vi "Get Test Skipped Message.vi"(8 "error in":errorcluster, 11 "Test In":refnum<class>) -> (0 "error out":errorcluster, 1 "IsTestCase":bool, 2 "skipMessage":string, 3 "Test Out":refnum<class>)   [LabVIEW 2013, in "TestResult.lvclass"]
uses:
  TestResult.lvclass
  TestCase/TestCase.lvclass
  TestSuite/TestSuite.lvclass
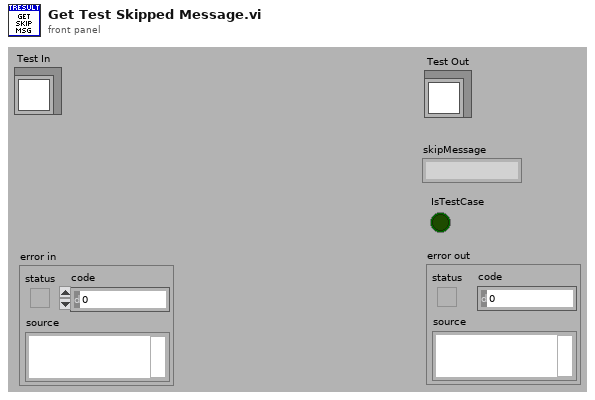
[diagram p1: front panel]
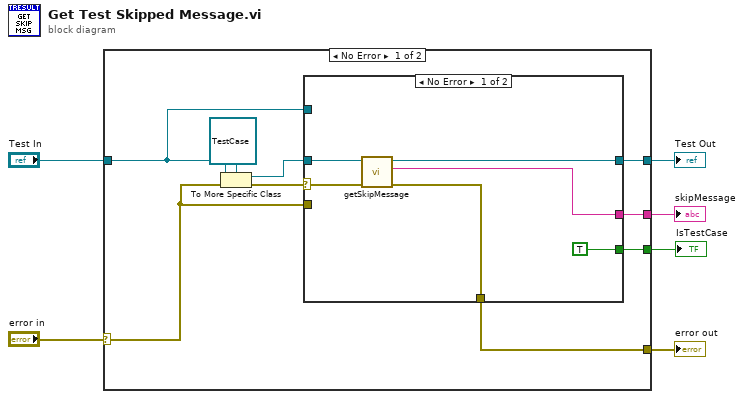
[diagram p0: block diagram]
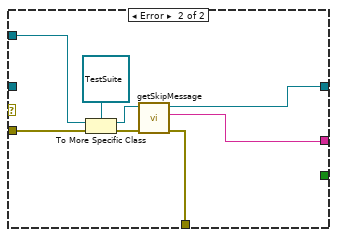
[diagram p2: hidden frame]
diagram:
  n1 = case shown="No Error" "error in" {
    selector: "error in" -> [w8 w31]
    tunnel: [w15 w31] -> w6
    tunnel: [w14 w30] -> w5
    tunnel: [w13 _] -> w4
    tunnel: "Test In" -> [w9 w30]
    tunnel: [w7 _] -> w1
    frame No Error {
      n2 = To More Specific Class(target class=refnum<class "TestCase.lvclass"> refnum ("TestCase.lvclass"), reference=w9, error in=w8) -> (specific class reference=w11:refnum<class "TestCase.lvclass">, error out=w12:errorcluster)
      n3 = case shown="No Error" w12 {
        selector: w12 -> [w17 _]
        tunnel: [w21 w22] -> w15
        tunnel: [w20 w23] -> w14
        tunnel: [w19 w24] -> w13
        tunnel: w11 -> [w18 _]
        tunnel: w8 -> [_ w28]
        tunnel: w9 -> [_ w27]
        tunnel: [TRUE ("IsTestCase") _] -> w7
        frame No Error {
          n4 = call-dynamic "getSkipMessage.vi"("error in (no error)"=w17, "TestCase in"=w18) -> ("error out"=w21:errorcluster, "skipMessage"=w19:string, "TestCase out"=w20:refnum<class "TestCase.lvclass">)  [unwired: 7 in]
        }
        frame Error {
          n5 = To More Specific Class(target class=refnum<class "TestSuite.lvclass"> refnum ("TestSuite.lvclass"), reference=w27, error in=w28) -> (specific class reference=w25:refnum<class "TestSuite.lvclass">, error out=w26:errorcluster)
          n6 = call-dynamic "getSkipMessage.vi"("error in (no error)"=w26, "TestSuite in"=w25) -> ("error out"=w22:errorcluster, "skipMessage"=w24:string, "TestSuite out"=w23:refnum<class "TestSuite.lvclass">)  [unwired: 7 in]
        }
      }
    }
    frame Error {
    }
  }
  "error out" <- w6
  "Test Out" <- w5
  "skipMessage" <- w4
  "IsTestCase" <- w1
